vi "Remove Panel.vi"(8 "error in (no error)":errorcluster, 10 "Panel":refnum<class "Panel.lvclass">, 11 "PanelArray in":refnum<class "PanelArray.lvclass">) -> (0 "error out":errorcluster, 3 "PanelArray out":refnum<class "PanelArray.lvclass">)   [LabVIEW 2018, in "OOPanel.lvlib" / "PanelArray.lvclass"]
uses:
  PanelArray.lvclass
  Panel/Panel.lvclass
  PanelArray.lvclass/PanelArray.ctl
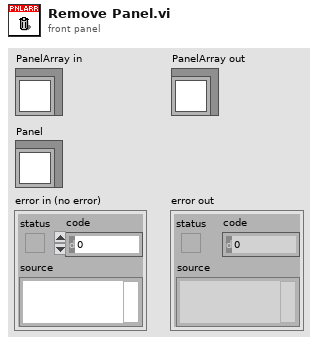
[diagram p1: front panel]
types:
  T1 = typedef "OOPanel.lvlib/PanelArray.lvclass/Ref Data.ctl" = cluster{"State":T2, "Refs":T3, "Events":T4, "Scrolling":T5, "Panels":T6}
  T2 = typedef "OOPanel.lvlib/PanelArray.lvclass/State.ctl" = cluster{"Defer Updates":bool, "Running":bool, "Dynamic Sizing":bool, "Borders":bool}
  T3 = typedef "OOPanel.lvlib/PanelArray.lvclass/Refs.ctl" = cluster{"SubPanels":refnum<vi>[], "Scrollbar":refnum<vi>, "Owning Panel":refnum<vi>}
  T4 = typedef "OOPanel.lvlib/PanelArray.lvclass/Events.ctl" = cluster{"Close":refnum<user-event>}
  T5 = typedef "OOPanel.lvlib/PanelArray.lvclass/Scrolling.ctl" = cluster{"Size":i32, "Max":i32, "Current":i32, "Top Index":i32, "Heights":i32[]}
  T6 = typedef "OOPanel.lvlib/PanelArray.lvclass/Panels.ctl" = cluster{"All":refnum<class "Panel.lvclass">[], "Visible":refnum<class "Panel.lvclass">[], "Blank":refnum<class "ArrayBlank.lvclass">}
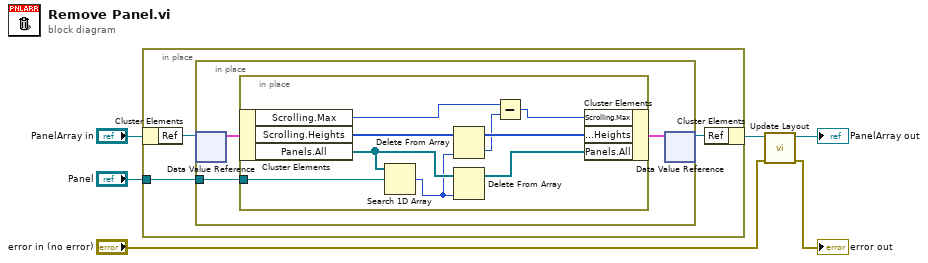
[diagram p0: block diagram]
diagram:
  n1 = in-place {
    in-place-border: "Panel" -> [w9]
    n2 = in-place-cluster #1("PanelArray in") -> ("Ref"=w8:refnum<data-value>)
    n3 = in-place {
      in-place-border: w9 -> [w12]
      n4 = in-place-dvr #2(w8) -> (w11:T1)  [unwired: 1 out]
      n5 = in-place {
        in-place-border: w12 -> [w13]
        n6 = in-place-cluster #3(w11) -> ("Scrolling.Max"=w17:i32, "Scrolling.Heights"=w20:i32[], "Panels.All"=w15:refnum<class "Panel.lvclass">[])
        n7 = Search 1D Array(1D array=w15, element=w13) -> (index of element=w14:i32)  [unwired: 1 in]
        n8 = Delete From Array(array=w20, index=w14) -> (deleted portion=w18:i32, array with subset deleted=w19:i32[])  [unwired: 1 in]
        n9 = Delete From Array(array=w15, index=w14) -> (array with subset deleted=w21:refnum<class "Panel.lvclass">[])  [unwired: 1 in, 1 out]
        n10 = Subtract(x=w17, y=w18) -> (x-y=w16:i32)
        n11 = in-place-cluster #3("Scrolling.Max"=w16, "Scrolling.Heights"=w19, "Panels.All"=w21) -> (w10:T1)
      }
      n12 = in-place-dvr #2(w10) -> (w7:refnum<data-value>)  [unwired: 1 out]
    }
    n13 = in-place-cluster #1("Ref"=w7) -> (w6:refnum<class "PanelArray.lvclass">)
  }
  n14 = call "Update Layout.vi"("error in (no error)"="error in (no error)", "PanelArray in"=w6) -> ("error out"=→"error out":errorcluster, "PanelArray out"=→"PanelArray out":refnum<class "PanelArray.lvclass">)  [unwired: 8 in]
